vi "espaciode_estados.vi"(2 "entrada u(t)":dbl=30.0, 3 "matriz C":dbl[](array[numeric])=[1.0, 0.0, 0.0], 4 "matriz B":dbl[](array[numeric])=[1.0, 0.0, 0.0], 5 "matriz  A":T1=[[0.0, 1.0, 0.0], [0.0, 0.0, 1.0], [-0.5, -4.0, -0.8]]) -> (0 "salida y(t)":dbl=5.620985756026012e+41 format="%.2f", 1 "x(K)":dbl[](array[numeric])=[5.620985756026012e+41, -2.4343062063073066e+42, 1.0542362075394749e+43])   [LabVIEW 2019]
doc: "Muestra el comportamiento solo de sistemas discretos representados en el espacio de estados apartir de una Matriz A y dos vectores B y C y con una entrada U(k)"
uses:
  <vilib>/Analysis/Matrix/Datatypes/RealMatrix.ctl
  <vilib>/Analysis/baseanly.llb/Real Dot Product.vi
  <vilib>/Analysis/baseanly.llb/A x Vector.vi
  <vilib>/Analysis/NI_AALBase.lvlib
  <vilib>/Analysis/Matrix/NI_Matrix.lvlib
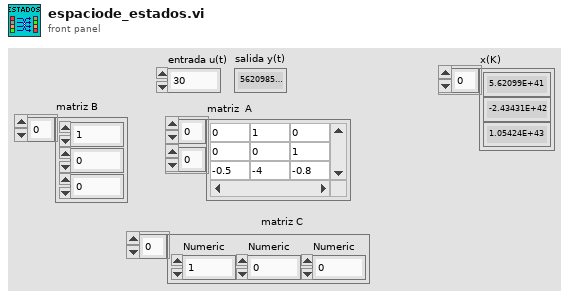
[diagram p1: front panel]
types:
  T1 = typedef "NI_Matrix.lvlib/RealMatrix.ctl" = dbl[][]
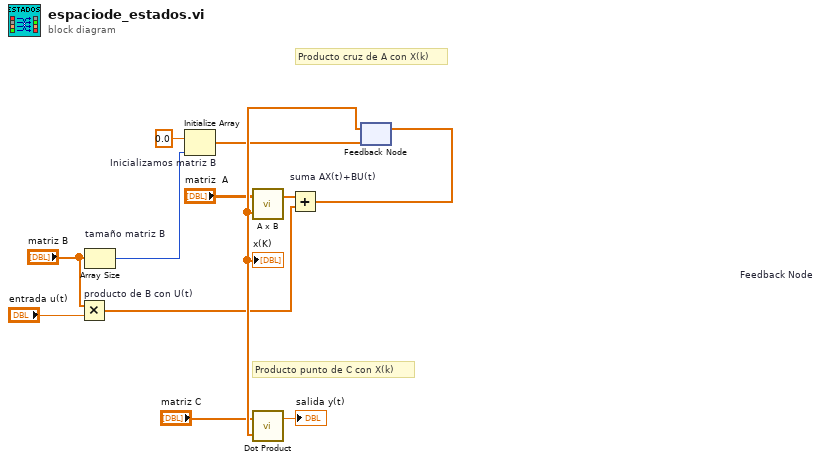
[diagram p0: block diagram]
diagram:
  # "Producto cruz de A con X(k)"
  # "Producto punto de C con X(k)"
  n1 = Multiply "producto de B con U(t)"(x="matriz B", y="entrada u(t)") -> (x*y=w4:dbl[])
  n2 = Array Size "tamaño matriz B"(array="matriz B") -> (size(s)=w8:i32)
  n3 = Initialize Array "Inicializamos matriz B"(0.0 ("element"), w8) -> (w10:dbl[])
  n4 = feedback #1 "Feedback Node"(w10) -> (w12:dbl[])
  "x(K)" <- w12
  n5 = call-poly <vilib>:"A x B.vi"("Vector"=w12, "A"="matriz  A") -> ("A x Vector"=w3:dbl[])  [unwired: 1 out]
  n6 = call-poly <vilib>:"Dot Product.vi"("Y Vector"=w12, "X Vector"="matriz C") -> ("X * Y"=→"salida y(t)":dbl)  [unwired: 1 out]
  n7 = Add "suma AX(t)+BU(t)"(x=w3, y=w4) -> (x+y=w11:dbl[])
  n8 = feedback-in #1(w11) -> ()
